vi "Home Page.vi"(11 "Error In":errorcluster) -> (4 "Home Msg":string="Home Message", 15 "Error Out":errorcluster)   [LabVIEW 2020, in "Sample Test Template.lvclass"]
doc: "Home page template"
uses:
  Sample Test Template.lvclass
  Typedef/User event controls.ctl
  ADC DAC Test Measurement.lvlib
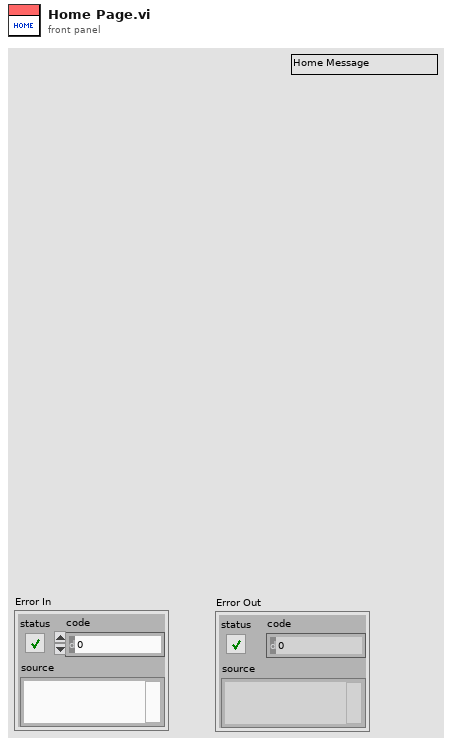
[diagram p1: front panel]
types:
  T1 = typedef "ADC DAC Test Measurement.lvlib/User event controls.ctl" = enum16{"Create", "Generate", "Run Test", "Get Ref", "Destroy"}
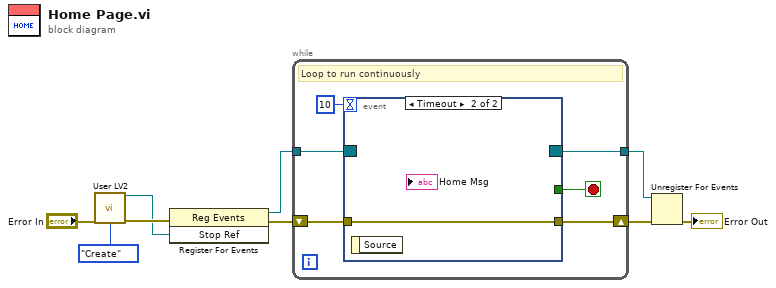
[diagram p0: block diagram]
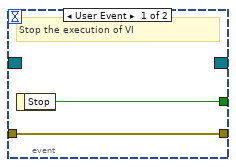
[diagram p2: hidden frame]
diagram:
  n1 = call "User LV2.vi"("Error In"="Error In", "User event controls"=User_event_controls."Create") -> ("Stop Ref"=w5:refnum<user-event>, "Error Out"=w7:errorcluster)  [unwired: 11 in, 1 out]
  n2 = register-events(error in=w7, w5) -> (reference out=w9:refnum<event-registration>, error out=w4:errorcluster)  [unwired: 1 in]
  n3 = while {
    tunnel: w9 -> [w15]
    tunnel: [w13] -> w2
    shift-right: [w11] -> w3
    shift-left: w4 -> [w12]
    stop <- w14 stop-if-true
    # "Loop to run continuously"
    n4 = event shown="[1] Timeout" {
      selector: w15 -> [_ _]
      dyn-events: [_ _] -> w13
      timeout: 10 -> [_ _]
      tunnel: [w17 _] -> w14
      tunnel: [w16 w18] -> w11
      tunnel: w12 -> [w16 w18]
      event User Event {
        # "Stop the execution of VI"
        n5 = event-data() -> ("Stop"=w17:bool)  [unwired: 1 in]
      }
      event Timeout {
        n6 = event-data() -> ()  [unwired: 1 in, 1 out]
      }
    }
  }
  n7 = Unregister For Events(event registration refnum=w2, error in=w3) -> (error out=→"Error Out":errorcluster)
